vi "BlueSimpleReachTask catch trial.vi"() -> ()   [LabVIEW 2010]
uses:
  Controls/Bits to Write.ctl
panel:
  in  "Arm Freeze Counter":bool
  in  "Time to wait\nbefore treat \nArm freeze (S)":dbl
  in  "Catch probability":i32=5 min=0 max=100 step=1
  out "Catch Trial?":bool
  out "DO Task":refnum<k21>="BlueSimple_DO_All"
  out "DI Task":refnum<k21>="BlueSimple_DI"
  out "Exp correct":i32
  out "Record flag":bool
  in  "Recenter motor":bool
  in  "Override bumps":bool
  in  "Start bump timer?":bool
  in  "Trial type":u16(ring) items=["Allflash/sensory", "Precue/memory"]
  in  "DBS On?":bool
  in  "Home+target OK?":bool
  out "Exp reset":bool
  out "target set #":i32
  in  "duration (s)":dbl=0.18 format="%.4f"
  in  "Inter-pulse delay":cluster{"Fix":dbl, "Rnd":dbl}={"Fix"=0.0, "Rnd"=1.5} {"Rnd" format="%.4f"; "Fix" format="%_4g"}
  in  "Autofeed?":bool
  out "Just initialized\nhold loop?":bool
  in  "Home reward?":bool
  in  "Home reward":cluster{"Fix":dbl, "Rnd":dbl} {"Rnd" format="%.4f"; "Fix" format="%_4g"}
  in  "Override 4":bool caption="Override 1"
  in  "Override 3":bool caption="Override 1"
  in  "Override 2":bool=TRUE caption="Override 1"
  in  "Override 1":bool=TRUE
  in  "LED lines":T1={"LED1"=1, "LED2"=2, "LED3"=3, "LED4"=4}
  in  "LED1":i16=5
  in  "LED2":i16=6
  in  "LED3":i16=7
  in  "LED4":i16=8
  in  "Bump Parameters":T2={"Distance (deg)"=2.0, "Travel time (ms)"=500.0} {"Travel time (ms)" min=0.1 max=10000.0; "Distance (deg)" min=0.1}
  in  "Bump delay":cluster{"Fix":dbl, "Rnd":dbl}={"Fix"=2.0, "Rnd"=8.0} {"Rnd" format="%.4f"; "Fix" format="%_4g"}
  in  "Sine parameters":T3={"Frequency"=1.0, "Degrees\npk-pk"=8.0, "Cycles"=10000} {"Degrees\npk-pk" min=0.1 max=120.0; "Frequency" min=0.001 format="%#_4g"}
  in  "Home":bool
  in  "Bumps":bool
  in  "Sines?":bool
  out "target set size":i32
  out "# target sets":u16
  in  "# Cycles":i16=20
  out "Instruct duration":dbl format="%.4f"
  out "Pre-I hold":dbl format="%.4f"
  out "Touching target\nlast time?":bool
  in  "Rand/Seq?":bool=TRUE
  in  "Target set":i16[](array[ring]) items=["1", "2", "3", "4"]
  in  "Block":T4(array[cluster])
  in  "Settings In":T5={"Pre-I hold"={"Fixed (s)"=0.5, "Random (s)"=0.5}, "LED I duration"={"Fixed (s)"=0.5, "Random (s)"=0.0}, "All Flash?"=FALSE, "Pre-cue brightness"=0, "Post-I hold"={"Fixed (s)"=0.7, "Random (s)"=0.3}, "Post-I \nbounce-off"={"Fixed (s)"=0.3, "Random (s)"=0.0}, "Capture timeout"={"Fixed (s)"=1.5, "Random (s)"=0.0}, "Tone duration"={"Fixed (s)"=0.5, "Random (s)"=0.0}, "LED C duration"={"Fixed (s)"=0.5, "Random (s)"=0.0}, "Cue brightness"=0, "Hold duration"={"Fixed (s)"=0.3, "Random (s)"=0.0}, "Allowed\nbounce-off"={"Fixed (s)"=0.2, "Random (s)"=0.0}, "Post-capture brightness"=0, "Reward duration"={"Fixed (s)"=0.7, "Random (s)"=0.0}, "Intertrial interval"={"Fixed (s)"=0.5, "Random (s)"=0.0}, "Persistent Mode?"=FALSE, "Error bong?"=TRUE, "Critter"=0, "Blocks"=[], "Target set"=[], "Rand/Seq?"=TRUE, "Trial type"=0, "Sines?"=FALSE, "Bumps"=FALSE, "Sine parameters"={"Frequency"=0.25, "Degrees\npk-pk"=6.0, "Cycles"=10000}, "Bump timing"={"Fix"=2.0, "Rnd"=8.0}, "Bump Parameters"={"Distance (deg)"=2.0, "Travel time (ms)"=500.0}, "DBS On?"=FALSE, "Home reward?"=FALSE, "Home+target OK?"=FALSE} {"Bump Parameters"."Travel time (ms)" min=0.1 max=10000.0; "Bump Parameters"."Distance (deg)" min=0.1; "Bump timing"."Rnd" format="%.4f"; "Bump timing"."Fix" format="%_4g"; "Sine parameters"."Degrees\npk-pk" min=0.1 max=120.0; "Sine parameters"."Frequency" min=0.001 format="%#_4g"; "Trial type" items=["Allflash/sensory", "Precue/memory"]; "Target set" items=["1", "2", "3", "4"]; "Critter" items=["Mojo", "Smokey"]; "Post-I \nbounce-off"."Random (s)" format="%.4f"; "Post-I \nbounce-off"."Fixed (s)" format="%_4g"; "Allowed\nbounce-off"."Random (s)" format="%.4f"; "Allowed\nbounce-off"."Fixed (s)" format="%_4g"; "LED C duration"."Random (s)" format="%.4f"; "LED C duration"."Fixed (s)" format="%.4f"; "Capture timeout"."Random (s)" format="%.4f"; "Capture timeout"."Fixed (s)" format="%.4f"; "Post-I hold"."Random (s)" format="%.4f"; "Post-I hold"."Fixed (s)" format="%.4f"; "Hold duration"."Random (s)" format="%.4f"; "Hold duration"."Fixed (s)" format="%_4g"; "Intertrial interval"."Random (s)" format="%.4f"; "Intertrial interval"."Fixed (s)" format="%.4f"; "Reward duration"."Random (s)" format="%.4f"; "Reward duration"."Fixed (s)" format="%.4f"; "LED I duration"."Random (s)" format="%.4f"; "LED I duration"."Fixed (s)" format="%.4f"; "Tone duration"."Random (s)" format="%.4f"; "Tone duration"."Fixed (s)" format="%.4f"; "Pre-I hold"."Random (s)" format="%.4f"; "Pre-I hold"."Fixed (s)" format="%_4g"}
  in  "pause":bool
  out "Assign settings":bool
  out "current path":path
  out "next trial path":path
  in  "Critter":u16(ring) items=["Mojo", "Smokey", "Blue", "Odo", "Monk 5", "Monk 6", "Monk 7", "Monk 8", "Monk 9", "Monk 10"]
  out "Total incorrect":i32
  in  "Write Settings":bool
  in  "Read Settings":bool
  in  "All Flash?":bool
  in  "Post-capture brightness":i16 caption="Brightness"
  in  "Cue brightness":i16=6 caption="Brightness"
  in  "Pre-cue brightness":i16 caption="Brightness"
  out "Total correct":i32
  out "Total %":dbl
  out "Total trials":i32
  in  "Error\nbong?":bool=TRUE
  out "TS Home":bool
  out "TS 4":bool
  out "TS 3":bool
  out "TS 2":bool
  out "TS 1":bool
  out "Waveform Chart":T6(graph)
  out "Block trials":i32
  out "Block %":dbl
  in  "Reset\ncounters":bool
  in  "Post-I \nbounce-off":cluster{"Fix":dbl, "Rnd":dbl}={"Fix"=0.3, "Rnd"=0.0} caption="Allowed\nbounce-off" {"Rnd" format="%.4f"; "Fix" format="%_4g"}
  out "Exp trials":i32
  out "Exp %":dbl
  in  "Touch lines":T7={"Home touch"=0, "Touch 1"=1, "Touch 2"=2, "Touch 3"=3, "Touch 4"=4}
  out "Current stage":T8(ring)
  in  "Allowed\nbounce-off":cluster{"Fix":dbl, "Rnd":dbl}={"Fix"=0.2, "Rnd"=0.0} {"Rnd" format="%.4f"; "Fix" format="%_4g"}
  in  "LED C duration":cluster{"Fix":dbl, "Rnd":dbl}={"Fix"=0.5, "Rnd"=0.0} caption="LED duration" {"Rnd" format="%.4f"; "Fix" format="%.4f"}
  in  "Capture timeout":cluster{"Fix":dbl, "Rnd":dbl}={"Fix"=1.5, "Rnd"=0.0} caption="Response time" {"Rnd" format="%.4f"; "Fix" format="%.4f"}
  in  "Post-I hold":cluster{"Fix":dbl, "Rnd":dbl}={"Fix"=0.5, "Rnd"=0.5} {"Rnd" format="%.4f"; "Fix" format="%.4f"}
  out "Last trial successful?":bool
  in  "Persistent\n Mode?":bool
  in  "Touch 4":i16=4
  in  "Touch 3":i16=3
  in  "Touch 2":i16=2
  in  "Touch 1":i16=1
  in  "Home touch":i16
  in  "Hold duration":cluster{"Fix":dbl, "Rnd":dbl}={"Fix"=0.2, "Rnd"=0.0} {"Rnd" format="%.4f"; "Fix" format="%_4g"}
  out "Target":i16
  in  "stop":bool
  in  "device":i16=1
  in  "line direction map":i32=2147483616 format="%.0b"
  out "DIGIO task ID":u32 format="%.0x"
  out "error out":errorcluster
  in  "Intertrial interval":cluster{"Fix":dbl, "Rnd":dbl}={"Fix"=0.5, "Rnd"=0.0} {"Rnd" format="%.4f"; "Fix" format="%.4f"}
  in  "Reward duration":cluster{"Fix":dbl, "Rnd":dbl}={"Fix"=0.38, "Rnd"=0.1} {"Rnd" format="%.4f"; "Fix" format="%.4f"}
  in  "LED I duration":cluster{"Fix":dbl, "Rnd":dbl}={"Fix"=0.5, "Rnd"=0.0} caption="LED duration" {"Rnd" format="%.4f"; "Fix" format="%.4f"}
  in  "Tone duration":cluster{"Fix":dbl, "Rnd":dbl}={"Fix"=0.5, "Rnd"=0.0} {"Rnd" format="%.4f"; "Fix" format="%.4f"}
  in  "Pre-I hold":cluster{"Fix":dbl, "Rnd":dbl}={"Fix"=0.5, "Rnd"=0.5} {"Rnd" format="%.4f"; "Fix" format="%_4g"}
  # "Auto-feed"
  # "DBS"
  # "Pre-\ninstruction\nhold"
  # "Post-\ninstruction\nhold"
  # "Instruction"
  # "Target capture"
  # "Target hold"
  # "Reward"
  # "Intertrial"
  # "Motor"
  # "Override"
  # "+"
  # "+"
  # "+"
  # "Pre-\ninstruction\nhold"
  # "Instruction"
  # "Post-\ninstruction\nhold"
  # "Target capture"
  # "Target hold"
  # "Reward"
  # "Intertrial"
  # "+"
  # "+"
  # "+"
  # "+"
  # "+"
  # "+"
  # "+"
  # "+"
  # "+"
  # "+"
  # "+"
  # "+"
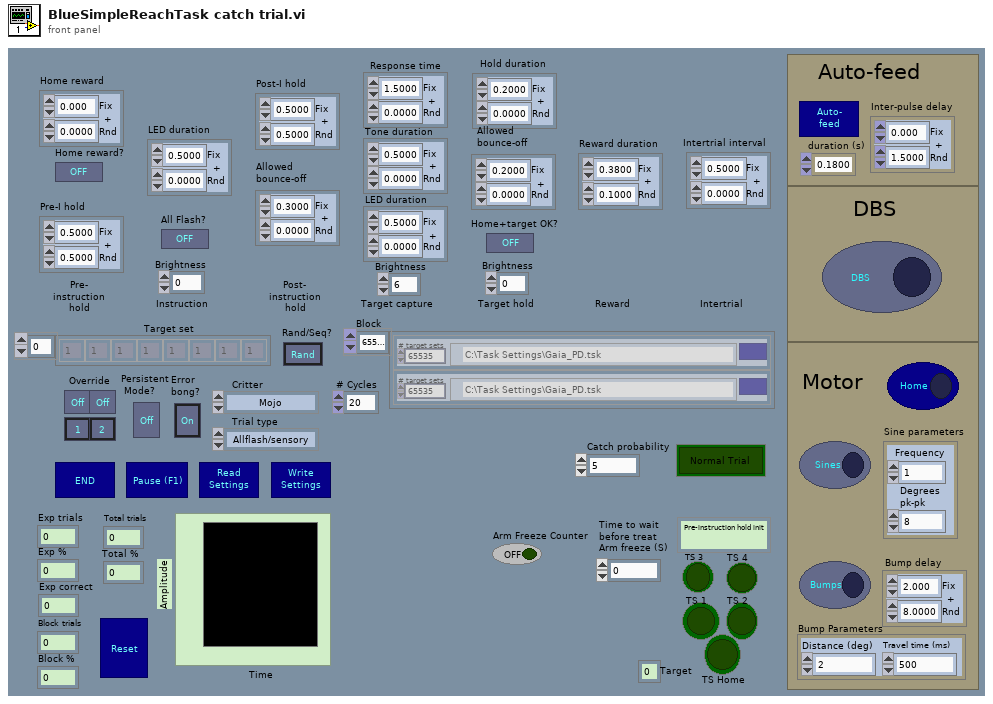
[diagram p1: front panel]
types:
  T1 = cluster{"LED1":i16, "LED2":i16, "LED3":i16, "LED4":i16}
  T2 = cluster{"Distance (deg)":dbl, "Travel time (ms)":dbl}
  T3 = cluster{"Frequency":dbl, "Degrees\npk-pk":dbl, "Cycles":i16}
  T4 = cluster{"Settings file":path, "# target sets":u16}[]
  T5 = cluster{"Pre-I hold":cluster{"Fixed (s)":dbl, "Random (s)":dbl}, "LED I duration":cluster{"Fixed (s)":dbl, "Random (s)":dbl}, "All Flash?":bool, "Pre-cue brightness":i16, "Post-I hold":cluster{"Fixed (s)":dbl, "Random (s)":dbl}, "Post-I \nbounce-off":cluster{"Fixed (s)":dbl, "Random (s)":dbl}, "Capture timeout":cluster{"Fixed (s)":dbl, "Random (s)":dbl}, "Tone duration":cluster{"Fixed (s)":dbl, "Random (s)":dbl}, "LED C duration":cluster{"Fixed (s)":dbl, "Random (s)":dbl}, "Cue brightness":i16, "Hold duration":cluster{"Fixed (s)":dbl, "Random (s)":dbl}, "Allowed\nbounce-off":cluster{"Fixed (s)":dbl, "Random (s)":dbl}, "Post-capture brightness":i16, "Reward duration":cluster{"Fixed (s)":dbl, "Random (s)":dbl}, "Intertrial interval":cluster{"Fixed (s)":dbl, "Random (s)":dbl}, "Persistent Mode?":bool, "Error bong?":bool, "Critter":u16, "Blocks":cluster{"Settings file":path, "# target sets":dbl}[], "Target set":i16[], "Rand/Seq?":bool, "Trial type":u16, "Sines?":bool, "Bumps":bool, "Sine parameters":cluster{"Frequency":dbl, "Degrees\npk-pk":dbl, "Cycles":i16}, "Bump timing":cluster{"Fix":dbl, "Rnd":dbl}, "Bump Parameters":cluster{"Distance (deg)":dbl, "Travel time (ms)":dbl}, "DBS On?":bool, "Home reward?":bool, "Home+target OK?":bool}
  T6 = cluster{"Segment Percentage":dbl, "Total % correct":dbl}
  T7 = cluster{"Home touch":i16, "Touch 1":i16, "Touch 2":i16, "Touch 3":i16, "Touch 4":i16}
  T8 = enum16{"Pre-instruction hold init", "Pre-instruction hold", "Instruction init", "Instruction", "Post-instruction hold init", "Post-instruction hold", "Target capture init", "Target capture", "Target hold init", "Target hold", "Reward stage", "Intertrial"}
  T9 = typedef "Bits to Write.ctl" = enum16{"LED 1 on", "LED 1 off", "LED 2 on", "LED 2 off", "LED 3 on", "LED 3 off", "LED 4 on", "LED 4 off", "All LEDs on", "All LEDs off", "In trial on", "In trial off", "Buzzer on", "Buzzer off", "Reward on", "Reward off", "Target number", "Trial type preQ on", "Trial type preQ off", "Error on", "Error off", "Trial number", "DBS on", "DBS off", "Sine on", "Sine off", "All Bits On", "All Bits Off", "Init", "Specify mask/pattern"}
  T10 = enum16{"Reset", "Increment", "Reset for exp", "Initialize"}
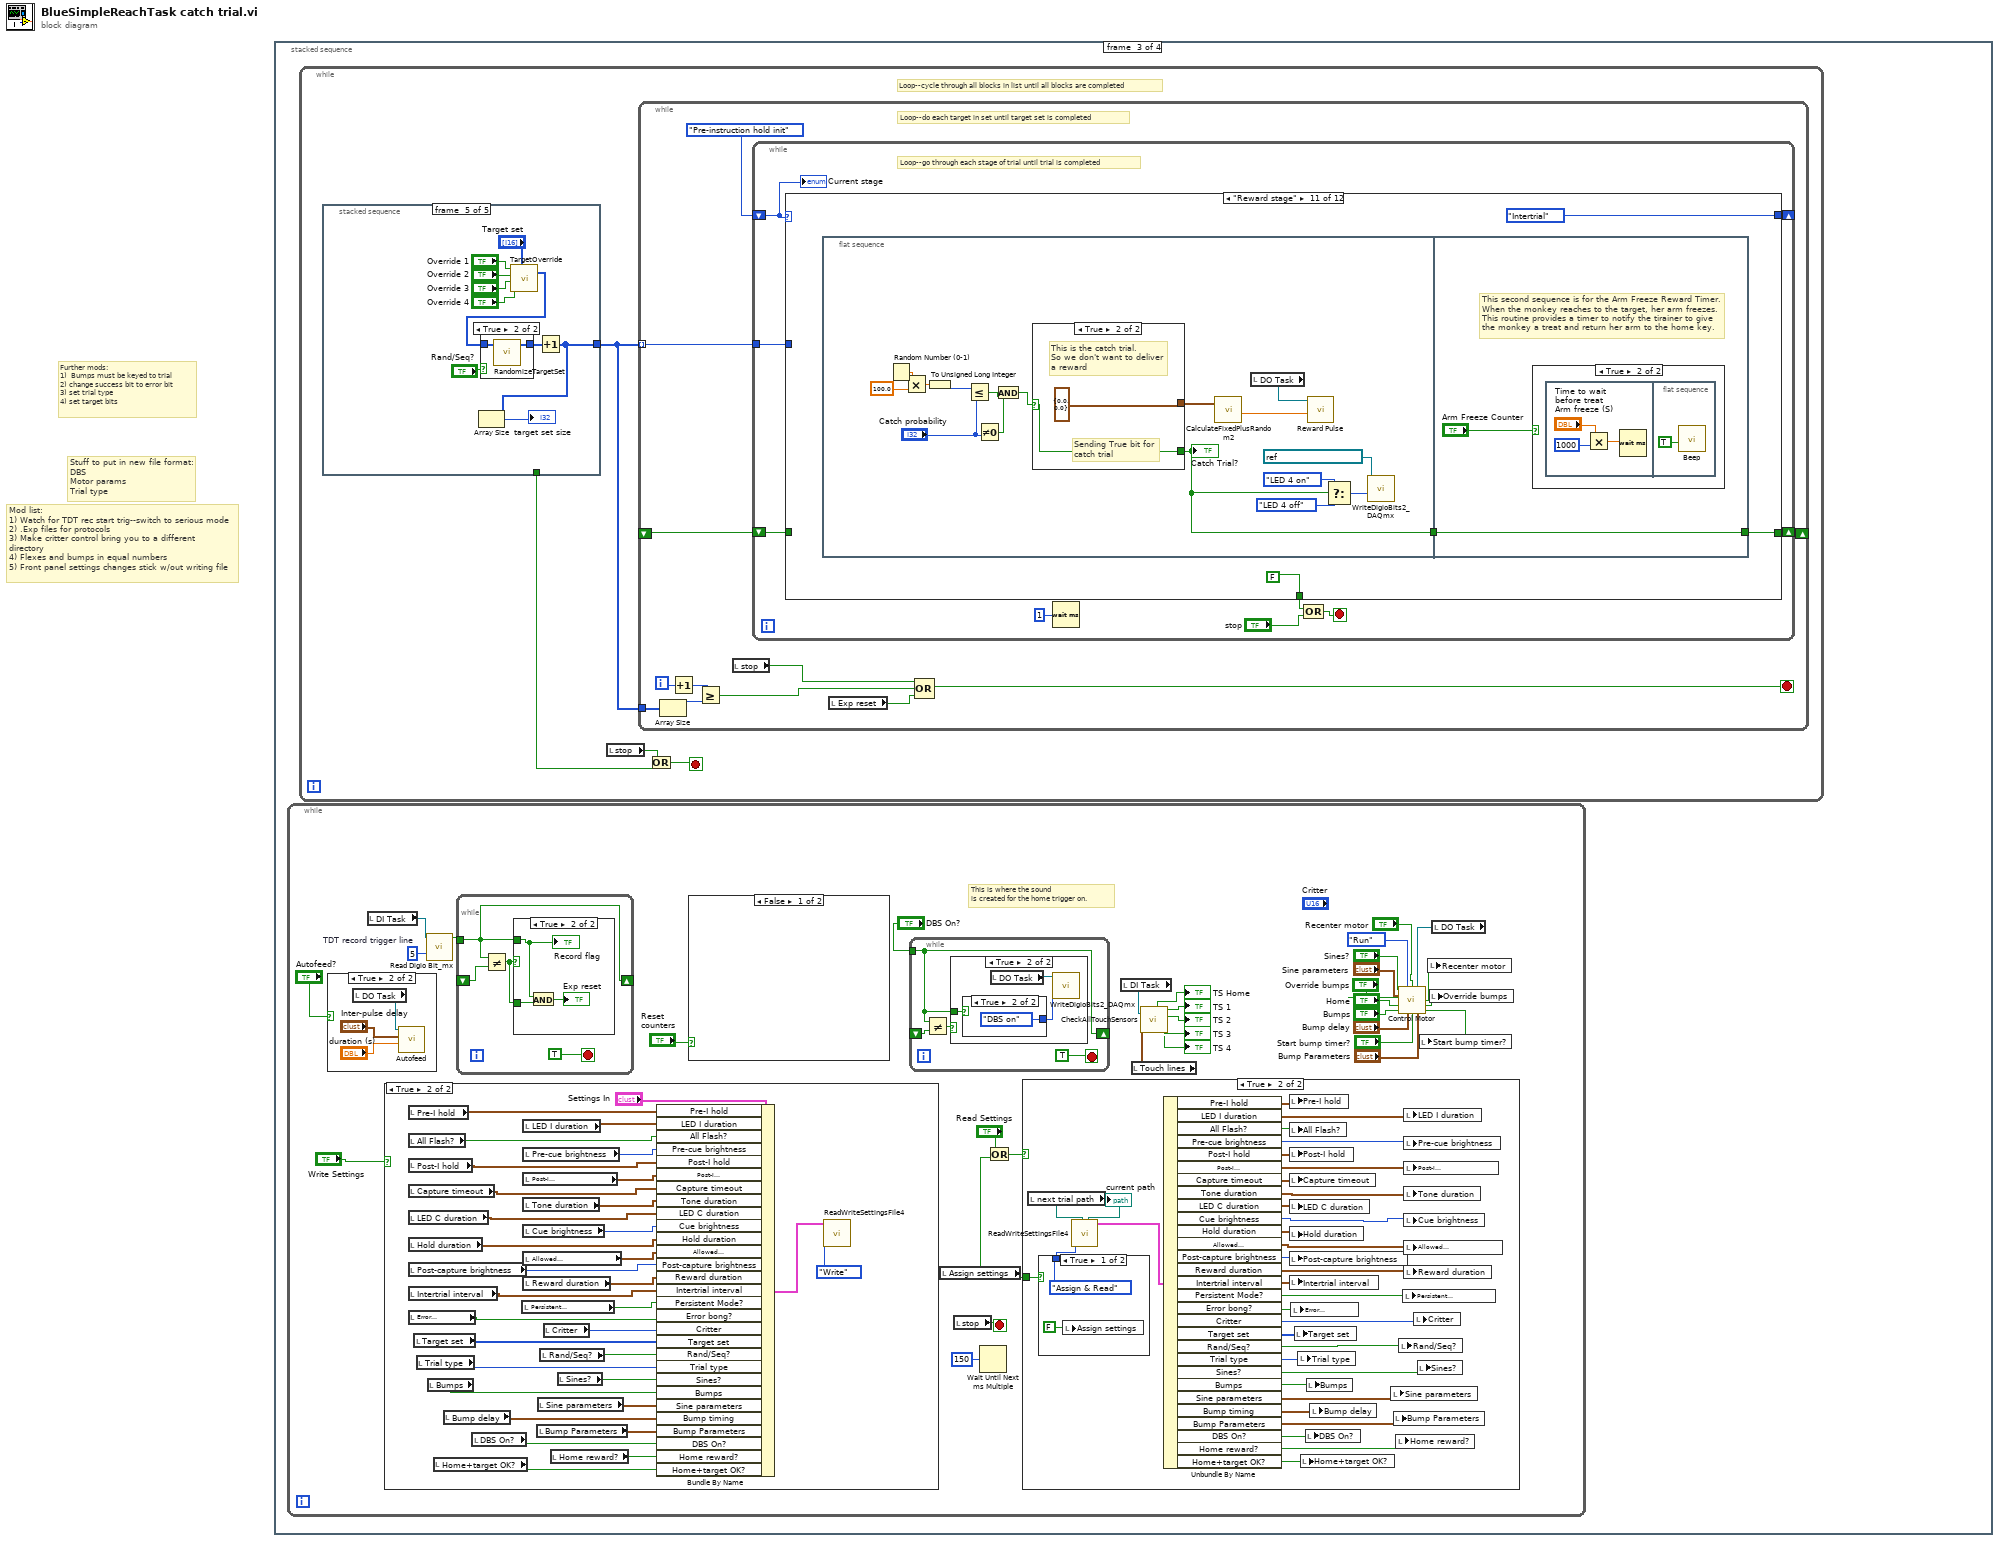
[diagram p0: block diagram]
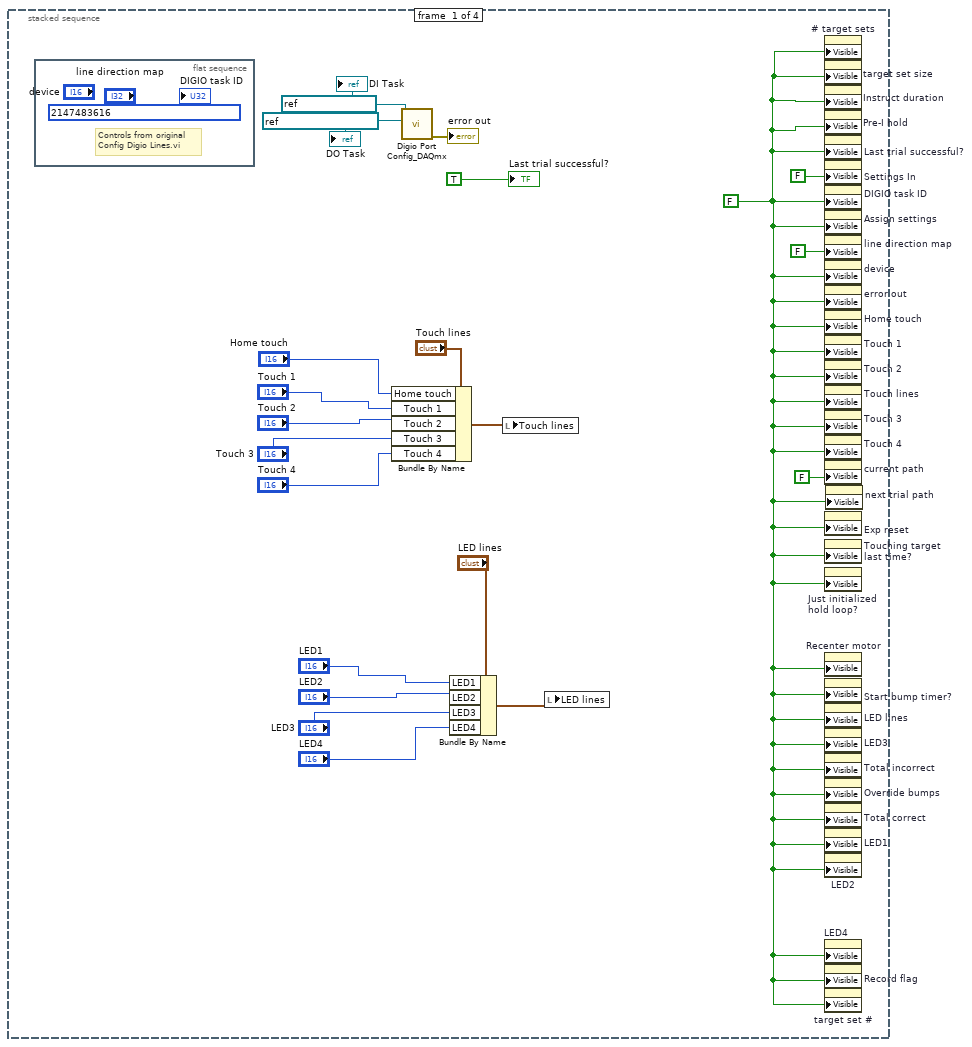
[diagram p2: hidden frame]
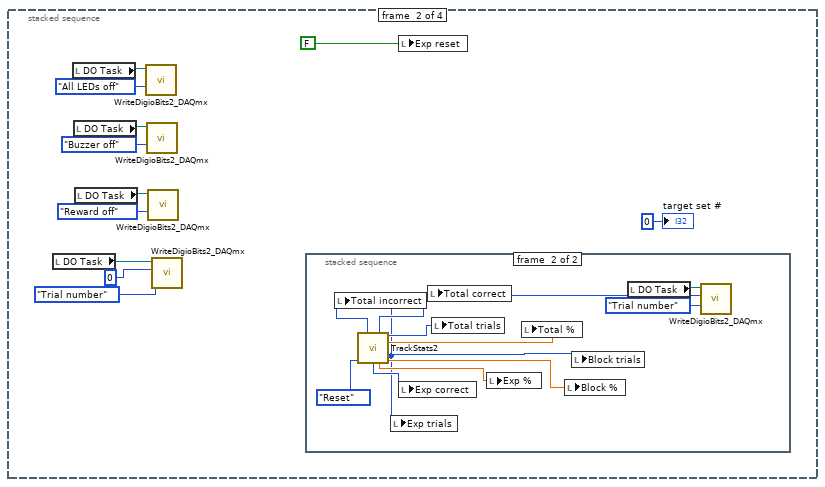
[diagram p3: hidden frame]
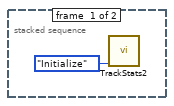
[diagram p4: hidden frame]
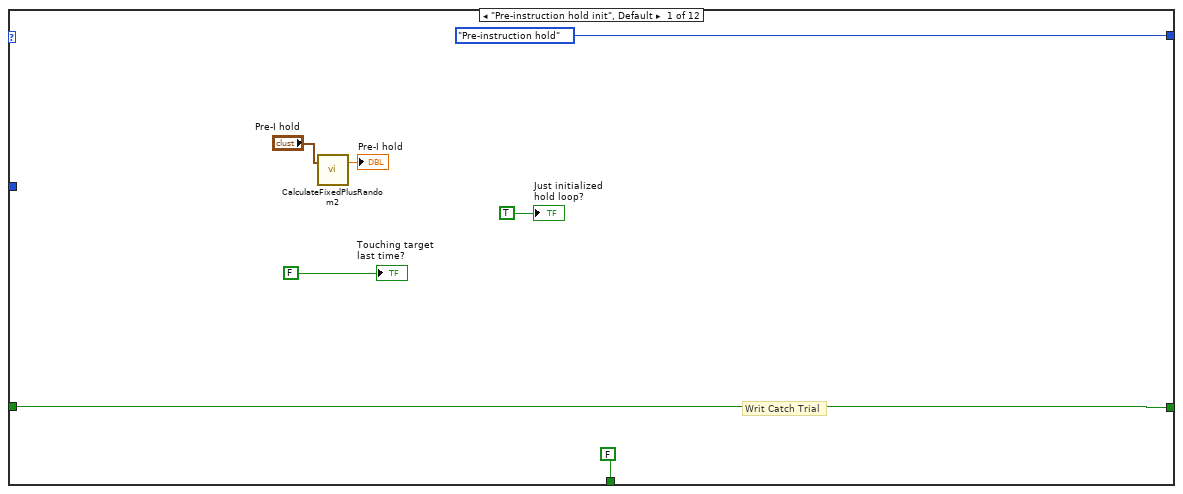
[diagram p5: hidden frame]
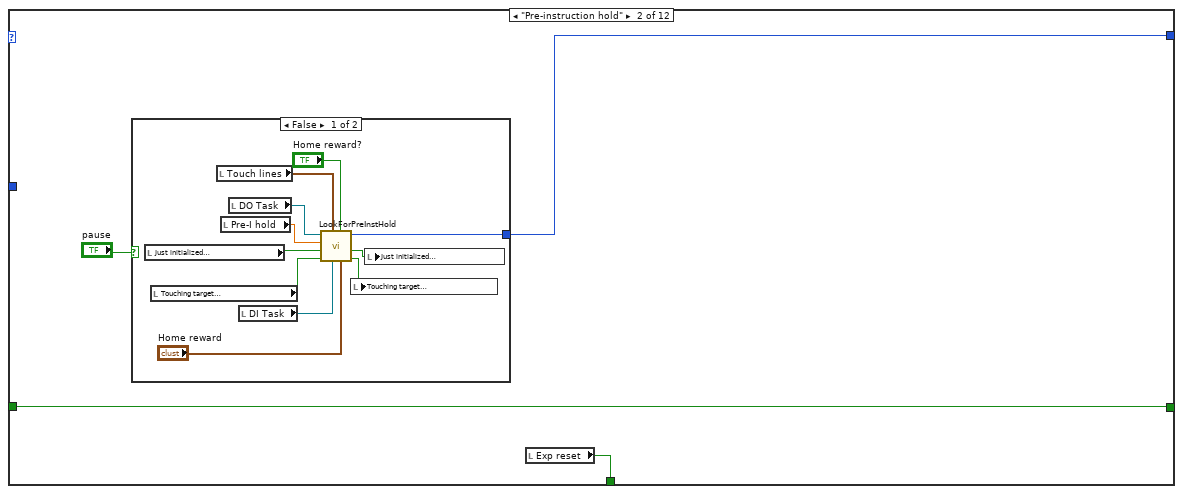
[diagram p6: hidden frame]
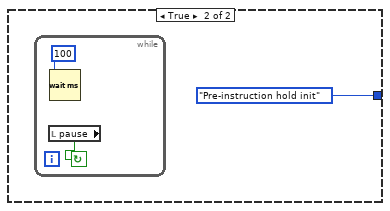
[diagram p7: hidden frame]
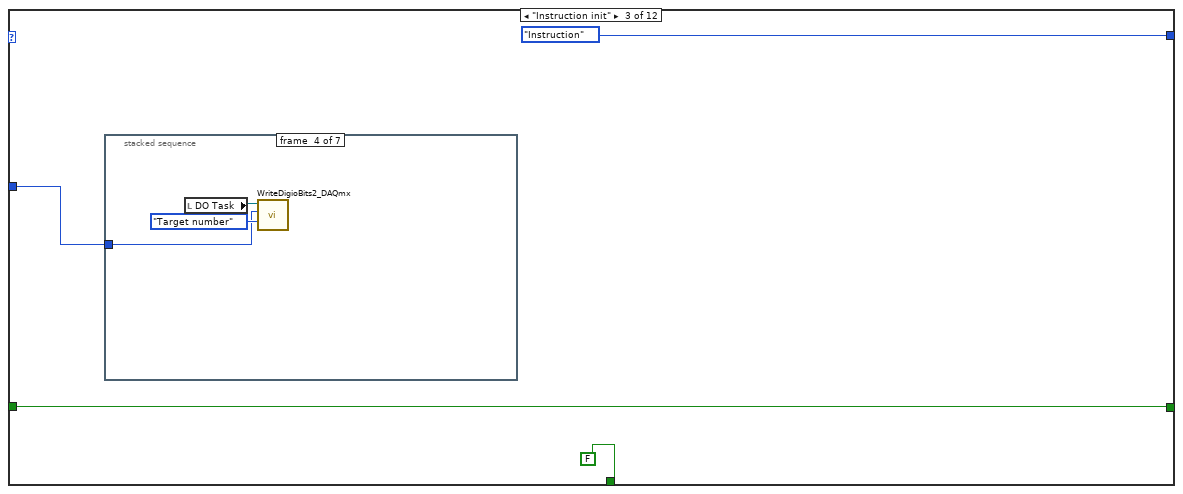
[diagram p8: hidden frame]
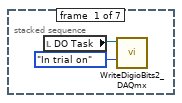
[diagram p9: hidden frame]
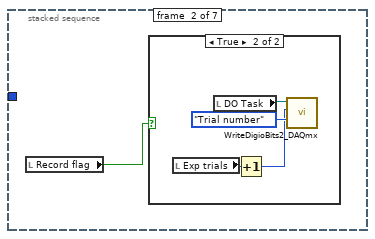
[diagram p10: hidden frame]
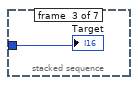
[diagram p12: hidden frame]
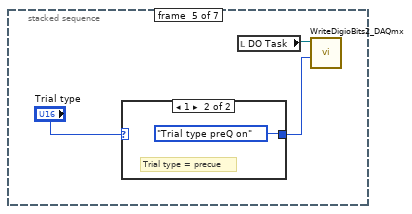
[diagram p13: hidden frame]
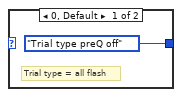
[diagram p14: hidden frame]
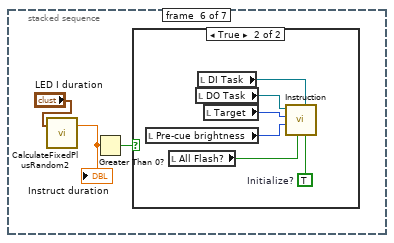
[diagram p15: hidden frame]
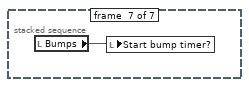
[diagram p17: hidden frame]
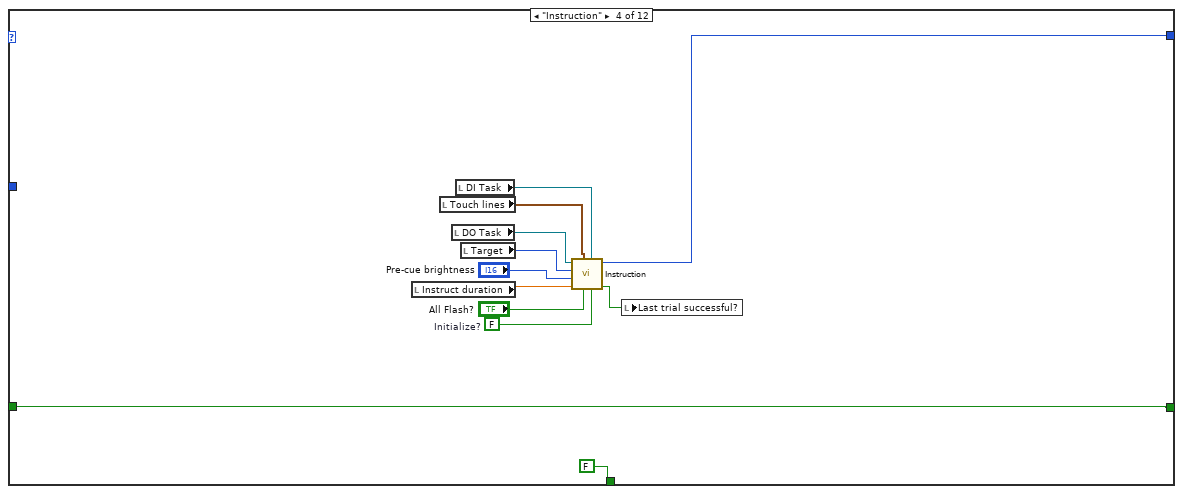
[diagram p18: hidden frame]
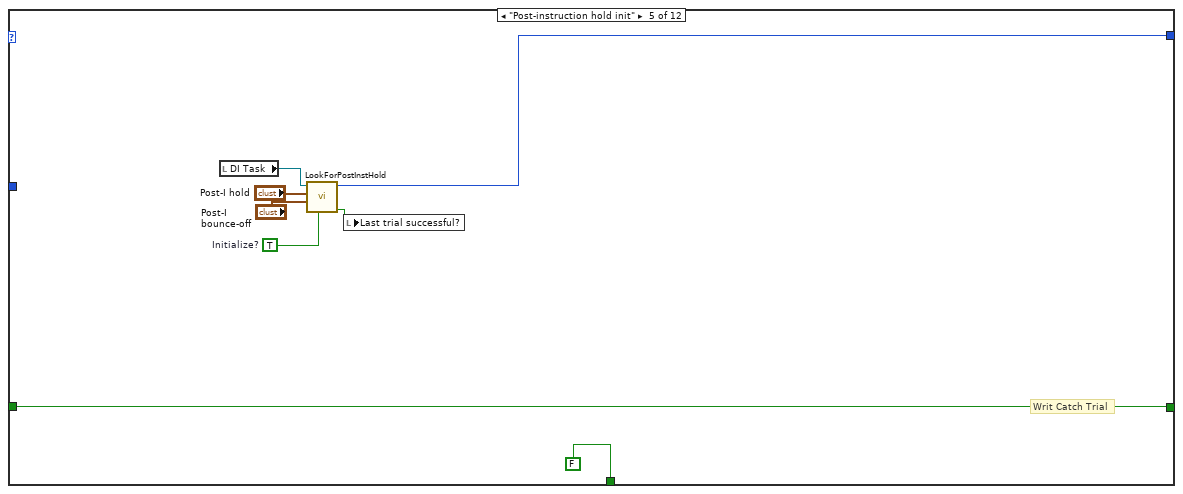
[diagram p19: hidden frame]
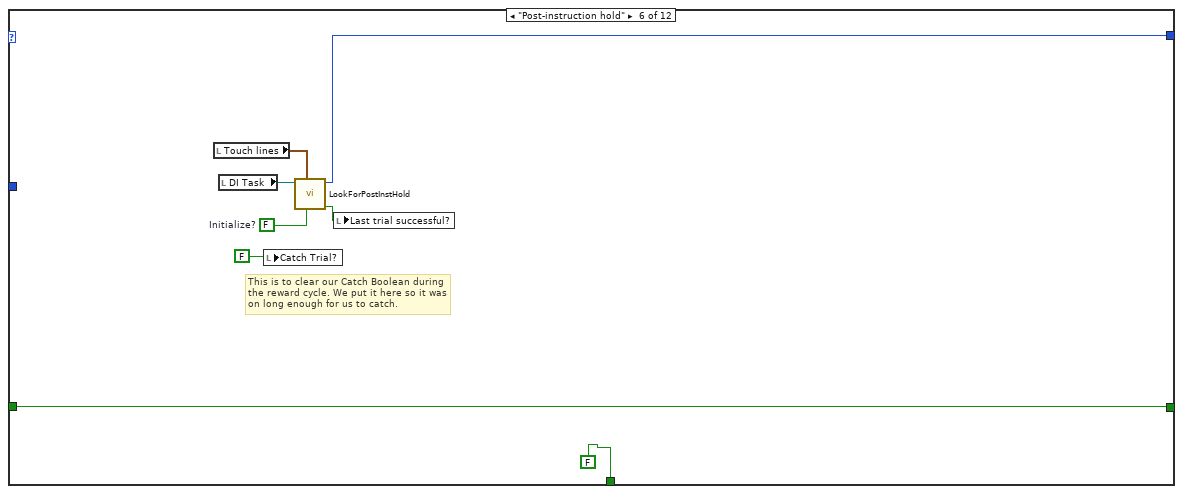
[diagram p20: hidden frame]
diagram:
  # "Stuff to put in new file format:\nDBS\nMotor params\nTrial type"
  # "Further mods:\n1)  Bumps must be keyed to trial\n2) change success bit to error bit\n3) set trial type\n4) set target bits"
  # "Mod list:\n1) Watch for TDT rec start trig--switch to serious mode\n2) .Exp files for protocols\n3) Make critter control bring you to a different directory\n4) Flexes and bumps in equal numbers\n5) Front panel settings changes stick w/out writing file"
  n1 = stacked-sequence {
    frame #0 {
      w2 = refnum<k21> "BlueSimple_DO_All" ("DO Task")
      w3 = refnum<k21> "BlueSimple_DI" ("DI Task")
      w4 = FALSE ("Persistent Mode?")
      n2 = flat-sequence {
        frame #0 {
          (unwired) 2147483616 ("line direction map")
          # "Controls from original\nConfig Digio Lines.vi"
        }
      }
      n3 = Bundle By Name(cluster="Touch lines", "Home touch"="Home touch", "Touch 1"="Touch 1", "Touch 2"="Touch 2", "Touch 3"="Touch 3", "Touch 4"="Touch 4") -> (w20:T7)
      n4 = call "Digio Port Config_DAQmx.vi"("DO Task"=w2, "DI Task"=w3) -> ("error out"=→"error out":errorcluster)  [unwired: 7 in]
      n5 = Bundle By Name(cluster="LED lines", "LED1"="LED1", "LED2"="LED2", "LED3"="LED3", "LED4"="LED4") -> (w8:T1)
      n6 = local write "Touch lines"(w20) -> ()
      n7 = local write "LED lines"(w8) -> ()
      n8 = property on="# target sets" class="DigNum (strict)"("Visible"=w4) -> ()  [unwired: 2 in, 2 out]
      n9 = property on="target set size" class="DigNum (strict)"("Visible"=w4) -> ()  [unwired: 2 in, 2 out]
      n10 = property on="Instruct duration" class="DigNum (strict)"("Visible"=w4) -> ()  [unwired: 2 in, 2 out]
      n11 = property on="Pre-I hold" class="DigNum (strict)"("Visible"=w4) -> ()  [unwired: 2 in, 2 out]
      n12 = property on="Last trial successful?" class="Bool (strict)"("Visible"=w4) -> ()  [unwired: 2 in, 2 out]
      n13 = property on="Settings In" class="Clust (strict)"("Visible"=FALSE) -> ()  [unwired: 2 in, 2 out]
      n14 = property on="DIGIO task ID" class="DigNum (strict)"("Visible"=w4) -> ()  [unwired: 2 in, 2 out]
      n15 = property on="Assign settings" class="Bool (strict)"("Visible"=w4) -> ()  [unwired: 2 in, 2 out]
      n16 = property on="line direction map" class="DigNum (strict)"("Visible"=FALSE) -> ()  [unwired: 2 in, 2 out]
      n17 = property on="device" class="DigNum (strict)"("Visible"=w4) -> ()  [unwired: 2 in, 2 out]
      n18 = property on="error out" class="Clust (strict)"("Visible"=w4) -> ()  [unwired: 2 in, 2 out]
      n19 = property on="Home touch" class="DigNum (strict)"("Visible"=w4) -> ()  [unwired: 2 in, 2 out]
      n20 = property on="Touch 1" class="DigNum (strict)"("Visible"=w4) -> ()  [unwired: 2 in, 2 out]
      n21 = property on="Touch 2" class="DigNum (strict)"("Visible"=w4) -> ()  [unwired: 2 in, 2 out]
      n22 = property on="Touch lines" class="Clust (strict)"("Visible"=w4) -> ()  [unwired: 2 in, 2 out]
      n23 = property on="Touch 3" class="DigNum (strict)"("Visible"=w4) -> ()  [unwired: 2 in, 2 out]
      n24 = property on="Touch 4" class="DigNum (strict)"("Visible"=w4) -> ()  [unwired: 2 in, 2 out]
      n25 = property on="current path" class="Path"("Visible"=FALSE) -> ()  [unwired: 2 in, 2 out]
      n26 = property on="Exp reset" class="Bool (strict)"("Visible"=w4) -> ()  [unwired: 2 in, 2 out]
      n27 = property on="Touching target\nlast time?" class="Bool (strict)"("Visible"=w4) -> ()  [unwired: 2 in, 2 out]
      n28 = property on="Just initialized\nhold loop?" class="Bool (strict)"("Visible"=w4) -> ()  [unwired: 2 in, 2 out]
      n29 = property on="Recenter motor" class="Bool (strict)"("Visible"=w4) -> ()  [unwired: 2 in, 2 out]
      n30 = property on="Start bump timer?" class="Bool (strict)"("Visible"=w4) -> ()  [unwired: 2 in, 2 out]
      n31 = property on="LED lines" class="Clust (strict)"("Visible"=w4) -> ()  [unwired: 2 in, 2 out]
      n32 = property on="LED3" class="DigNum (strict)"("Visible"=w4) -> ()  [unwired: 2 in, 2 out]
      n33 = property on="Total incorrect" class="DigNum (strict)"("Visible"=w4) -> ()  [unwired: 2 in, 2 out]
      n34 = property on="Override bumps" class="Bool (strict)"("Visible"=w4) -> ()  [unwired: 2 in, 2 out]
      n35 = property on="Total correct" class="DigNum (strict)"("Visible"=w4) -> ()  [unwired: 2 in, 2 out]
      n36 = property on="LED1" class="DigNum (strict)"("Visible"=w4) -> ()  [unwired: 2 in, 2 out]
      n37 = property on="LED2" class="DigNum (strict)"("Visible"=w4) -> ()  [unwired: 2 in, 2 out]
      n38 = property on="LED4" class="DigNum (strict)"("Visible"=w4) -> ()  [unwired: 2 in, 2 out]
      n39 = property on="Record flag" class="Bool (strict)"("Visible"=w4) -> ()  [unwired: 2 in, 2 out]
      n40 = property on="target set #" class="DigNum (strict)"("Visible"=w4) -> ()  [unwired: 2 in, 2 out]
      n41 = property on="next trial path" class="Path"("Visible"=w4) -> ()  [unwired: 2 in, 2 out]
      "Last trial successful?" <- TRUE ("Persistent Mode?")
      "DI Task" <- w3
      "DO Task" <- w2
    }
    frame #1 {
      n42 = local read "DO Task"() -> (w30:refnum<k21>)
      n43 = local read "DO Task"() -> (w23:refnum<k21>)
      n44 = local read "DO Task"() -> (w24:refnum<k21>)
      n45 = local read "DO Task"() -> (w26:refnum<k21>)
      n46 = call "WriteDigioBits2_DAQmx.vi"("Bits to write"=Bits_to_Write."All LEDs off", "DO Task"=w23) -> ()  [unwired: 9 in, 1 out]
      n47 = call "WriteDigioBits2_DAQmx.vi"("Bits to write"=Bits_to_Write."Buzzer off", "DO Task"=w24) -> ()  [unwired: 9 in, 1 out]
      n48 = call "WriteDigioBits2_DAQmx.vi"("Bits to write"=Bits_to_Write."Reward off", "DO Task"=w26) -> ()  [unwired: 9 in, 1 out]
      n49 = call "WriteDigioBits2_DAQmx.vi"("Bits to write"=Bits_to_Write."Trial number", "Number"=u32 0, "DO Task"=w30) -> ()  [unwired: 8 in, 1 out]
      n50 = stacked-sequence {
        frame #0 {
          n51 = call "TrackStats2.vi"("Command"=T10."Initialize") -> ()  [unwired: 6 in, 9 out]
        }
        frame #1 {
          n52 = call "TrackStats2.vi"("Command"=T10."Reset") -> ("Total incorrect"=w45:i32, "Total correct"=w44:i32, "# total trials"=w43:i32, "Total % correct"=w42:dbl, "Segment trials"=w38:i32, "Experiment trials"=w34:i32, "Experiment correct"=w37:i32, "Experiment %"=w40:dbl, "Segment Percentage"=w41:dbl)  [unwired: 6 in]
          n53 = local write "Total incorrect"(w45) -> ()
          n54 = local write "Exp trials"(w34) -> ()
          n55 = local write "Exp correct"(w37) -> ()
          n56 = local write "Total correct"(w44) -> ()
          n57 = local write "Total trials"(w43) -> ()
          n58 = local write "Exp %"(w40) -> ()
          n59 = local write "Total %"(w42) -> ()
          n60 = local write "Block %"(w41) -> ()
          n61 = local write "Block trials"(w38) -> ()
          n62 = local read "DO Task"() -> (w36:refnum<k21>)
          n63 = call "WriteDigioBits2_DAQmx.vi"("Bits to write"=Bits_to_Write."Trial number", "Number"=w34, "DO Task"=w36) -> ()  [unwired: 8 in, 1 out]
        }
      }
      n64 = local write "Exp reset"(FALSE ("Exp reset")) -> ()
      "target set #" <- 0 ("target set #")
    }
    frame #2 {
      n65 = while {
        stop <- w334 stop-if-true
        w305 = i16 5  # TDT record trigger line
        # "This is where the sound\nis created for the home trigger on."
        n66 = case shown="True" "Autofeed?" {
          frame False {
          }
          frame True {
            n67 = local read "DO Task"() -> (w344:refnum<k21>)
            n68 = call "Autofeed.vi"("duration"="duration (s)", "Auto-feed"="Inter-pulse delay", "DO Task"=w344) -> ()  [unwired: 4 in]
          }
        }
        n69 = local read "DI Task"() -> (w304:refnum<k21>)
        n70 = case shown="True" "Write Settings" {
          frame False {
          }
          frame True {
            n71 = local read "Pre-I hold"() -> (w385:cluster{"Fix":dbl, "Rnd":dbl})
            n72 = local read "All Flash?"() -> (w383:bool)
            n73 = local read "Post-I hold"() -> (w381:cluster{"Fix":dbl, "Rnd":dbl})
            n74 = local read "Capture timeout"() -> (w379:cluster{"Fix":dbl, "Rnd":dbl})
            n75 = local read "LED C duration"() -> (w377:cluster{"Fix":dbl, "Rnd":dbl})
            n76 = local read "Hold duration"() -> (w375:cluster{"Fix":dbl, "Rnd":dbl})
            n77 = local read "Post-capture brightness"() -> (w373:i16)
            n78 = local read "Intertrial interval"() -> (w371:cluster{"Fix":dbl, "Rnd":dbl})
            n79 = local read "Error\nbong?"() -> (w369:bool)
            n80 = local read "Target set"() -> (w365:i16[])
            n81 = local read "Trial type"() -> (w362:u16)
            n82 = local read "Bumps"() -> (w360:bool)
            n83 = local read "Home+target OK?"() -> (w354:bool)
            n84 = local read "Bump delay"() -> (w358:cluster{"Fix":dbl, "Rnd":dbl})
            n85 = local read "DBS On?"() -> (w356:bool)
            n86 = local read "Persistent\n Mode?"() -> (w370:bool)
            n87 = local read "LED I duration"() -> (w384:cluster{"Fix":dbl, "Rnd":dbl})
            n88 = local read "Pre-cue brightness"() -> (w382:i16)
            n89 = local read "Post-I \nbounce-off"() -> (w380:cluster{"Fix":dbl, "Rnd":dbl})
            n90 = local read "Tone duration"() -> (w378:cluster{"Fix":dbl, "Rnd":dbl})
            n91 = local read "Cue brightness"() -> (w376:i16)
            n92 = local read "Allowed\nbounce-off"() -> (w374:cluster{"Fix":dbl, "Rnd":dbl})
            n93 = local read "Reward duration"() -> (w372:cluster{"Fix":dbl, "Rnd":dbl})
            n94 = local read "Bump Parameters"() -> (w357:T2)
            n95 = local read "Sine parameters"() -> (w359:T3)
            n96 = local read "Rand/Seq?"() -> (w364:bool)
            n97 = local read "Critter"() -> (w366:u16)
            n98 = local read "Home reward?"() -> (w355:bool)
            n99 = local read "Sines?"() -> (w361:bool)
            n100 = Bundle By Name(cluster="Settings In", "Pre-I hold"=w385, "LED I duration"=w384, "All Flash?"=w383, "Pre-cue brightness"=w382, "Post-I hold"=w381, "Post-I \nbounce-off"=w380, "Capture timeout"=w379, "Tone duration"=w378, "LED C duration"=w377, "Cue brightness"=w376, "Hold duration"=w375, "Allowed\nbounce-off"=w374, "Post-capture brightness"=w373, "Reward duration"=w372, "Intertrial interval"=w371, "Persistent Mode?"=w370, "Error bong?"=w369, "Critter"=w366, "Target set"=w365, "Rand/Seq?"=w364, "Trial type"=w362, "Sines?"=w361, "Bumps"=w360, "Sine parameters"=w359, "Bump timing"=w358, "Bump Parameters"=w357, "DBS On?"=w356, "Home reward?"=w355, "Home+target OK?"=w354) -> (w363:T5)
            n101 = call "ReadWriteSettingsFile4.vi"("Read/write"=enum16{"Query & Read", "Assign & Read", "Write"}."Write", "Settings In"=w363) -> ()  [unwired: 4 in, 4 out]
          }
        }
        n102 = call "Read Digio Bit_mx.vi"("line"=w305, "DI Task"=w304) -> ("line state"=w303:bool)  [unwired: 7 in, 1 out]
        n103 = while {
          tunnel: w303 -> [w348]
          shift-right: [w348] -> _
          shift-left: _ -> [w349]
          stop <- TRUE stop-if-true
          n104 = Not Equal?(x=w348, y=w349) -> (x != y?=w347:bool)
          n105 = case shown="True" w347 {
            tunnel: w348 -> [_ w351]
            tunnel: w347 -> [_ w352]
            frame False {
            }
            frame True {
              n106 = And(x=w351, y=w352) -> (x .and. y?=→"Exp reset":bool)
              "Record flag" <- w351
            }
          }
        }
        n107 = case shown="False" "Reset\ncounters" {
          frame False {
          }
          frame True {
            n108 = call "TrackStats2.vi"("Command"=T10."Reset") -> ("Total incorrect"=w431:i32, "Total correct"=w430:i32, "# total trials"=w429:i32, "Total % correct"=w428:dbl, "Segment trials"=w427:i32, "Experiment trials"=w424:i32, "Experiment %"=w425:dbl, "Segment Percentage"=w426:dbl)  [unwired: 6 in, 1 out]
            n109 = local write "Total incorrect"(w431) -> ()
            n110 = local write "Total correct"(w430) -> ()
            n111 = local write "Exp trials"(w424) -> ()
            n112 = local write "Exp %"(w425) -> ()
            n113 = local write "Block %"(w426) -> ()
            n114 = local write "Block trials"(w427) -> ()
            n115 = local write "Total trials"(w429) -> ()
            n116 = local write "Total %"(w428) -> ()
          }
        }
        n117 = while {
          shift-right: [w336] -> _
          shift-left: _ -> [w337]
          tunnel: "DBS On?" -> [w336]
          stop <- TRUE stop-if-true
          n118 = Not Equal?(x=w336, y=w337) -> (x != y?=w335:bool)
          n119 = case shown="True" w335 {
            tunnel: w336 -> [_ w341]
            frame False {
            }
            frame True {
              n120 = case shown="True" w341 {
                tunnel: [Bits_to_Write."DBS off" ("Bits to write") Bits_to_Write."DBS on" ("Bits to write")] -> w339
                frame False {
                }
                frame True {
                }
              }
              n121 = local read "DO Task"() -> (w340:refnum<k21>)
              n122 = call "WriteDigioBits2_DAQmx.vi"("Bits to write"=w339, "DO Task"=w340) -> ()  [unwired: 9 in, 1 out]
            }
          }
        }
        n123 = local read "Assign settings"() -> (w323:bool)
        n124 = local read "stop"() -> (w334:bool)
        n125 = Wait Until Next ms Multiple(millisecond multiple=u32 150) -> ()  [unwired: 1 out]
        n126 = Or(x="Read Settings", y=w323) -> (x .or. y?=w324:bool)
        n127 = case shown="True" w324 {
          tunnel: w323 -> [_ w398]
          frame False {
          }
          frame True {
            n128 = local read "next trial path"() -> (w399:path)
            n129 = case shown="True" w398 {
              tunnel: [enum16{"Query & Read", "Assign & Read", "Write"}."Assign & Read" ("Read/write") enum16{"Query & Read", "Assign & Read", "Write"}."Query & Read" ("Read/write")] -> w401
              frame True {
                n130 = local write "Assign settings"(FALSE ("Assign settings")) -> ()
              }
              frame False {
              }
            }
            n131 = call "ReadWriteSettingsFile4.vi"("file path"=w399, "Read/write"=w401) -> ("Settings Out"=w419:T5, "current path"=→"current path":path)  [unwired: 4 in, 2 out]
            n132 = Unbundle By Name(w419) -> ("Pre-I hold"=w418:cluster{"Fixed (s)":dbl, "Random (s)":dbl}, "LED I duration"=w417:cluster{"Fixed (s)":dbl, "Random (s)":dbl}, "All Flash?"=w416:bool, "Pre-cue brightness"=w415:i16, "Post-I hold"=w414:cluster{"Fixed (s)":dbl, "Random (s)":dbl}, "Post-I \nbounce-off"=w413:cluster{"Fixed (s)":dbl, "Random (s)":dbl}, "Capture timeout"=w412:cluster{"Fixed (s)":dbl, "Random (s)":dbl}, "Tone duration"=w411:cluster{"Fixed (s)":dbl, "Random (s)":dbl}, "LED C duration"=w410:cluster{"Fixed (s)":dbl, "Random (s)":dbl}, "Cue brightness"=w409:i16, "Hold duration"=w408:cluster{"Fixed (s)":dbl, "Random (s)":dbl}, "Allowed\nbounce-off"=w407:cluster{"Fixed (s)":dbl, "Random (s)":dbl}, "Post-capture brightness"=w406:i16, "Reward duration"=w405:cluster{"Fixed (s)":dbl, "Random (s)":dbl}, "Intertrial interval"=w404:cluster{"Fixed (s)":dbl, "Random (s)":dbl}, "Persistent Mode?"=w403:bool, "Error bong?"=w402:bool, "Critter"=w397:u16, "Target set"=w396:i16[], "Rand/Seq?"=w395:bool, "Trial type"=w394:u16, "Sines?"=w393:bool, "Bumps"=w392:bool, "Sine parameters"=w391:T3, "Bump timing"=w390:cluster{"Fix":dbl, "Rnd":dbl}, "Bump Parameters"=w389:T2, "DBS On?"=w388:bool, "Home reward?"=w387:bool, "Home+target OK?"=w386:bool)
            n133 = local write "Pre-I hold"(w418) -> ()
            n134 = local write "All Flash?"(w416) -> ()
            n135 = local write "Post-I hold"(w414) -> ()
            n136 = local write "Capture timeout"(w412) -> ()
            n137 = local write "LED C duration"(w410) -> ()
            n138 = local write "Hold duration"(w408) -> ()
            n139 = local write "Post-capture brightness"(w406) -> ()
            n140 = local write "Intertrial interval"(w404) -> ()
            n141 = local write "Error\nbong?"(w402) -> ()
            n142 = local write "Target set"(w396) -> ()
            n143 = local write "Trial type"(w394) -> ()
            n144 = local write "Home+target OK?"(w386) -> ()
            n145 = local write "DBS On?"(w388) -> ()
            n146 = local write "Bumps"(w392) -> ()
            n147 = local write "Bump delay"(w390) -> ()
            n148 = local write "Sine parameters"(w391) -> ()
            n149 = local write "Bump Parameters"(w389) -> ()
            n150 = local write "Home reward?"(w387) -> ()
            n151 = local write "Rand/Seq?"(w395) -> ()
            n152 = local write "Persistent\n Mode?"(w403) -> ()
            n153 = local write "LED I duration"(w417) -> ()
            n154 = local write "Pre-cue brightness"(w415) -> ()
            n155 = local write "Post-I \nbounce-off"(w413) -> ()
            n156 = local write "Tone duration"(w411) -> ()
            n157 = local write "Cue brightness"(w409) -> ()
            n158 = local write "Allowed\nbounce-off"(w407) -> ()
            n159 = local write "Reward duration"(w405) -> ()
            n160 = local write "Critter"(w397) -> ()
            n161 = local write "Sines?"(w393) -> ()
          }
        }
        n162 = local read "DI Task"() -> (w332:refnum<k21>)
        n163 = local read "Touch lines"() -> (w331:T7)
        n164 = call "CheckAllTouchSensors.vi"("Touch sensor lines"=w331, "DI Task"=w332) -> ("TS 4"=→"TS 4":bool, "TS 3"=→"TS 3":bool, "TS 2"=→"TS 2":bool, "TS 1"=→"TS 1":bool, "Home?"=→"TS Home":bool)
        n165 = local read "DO Task"() -> (w306:refnum<k21>)
        n166 = call "Control Motor.vi"("Sines?"="Sines?", "Command"=enum16{"Initialize", "Home", "Run", "Disable"}."Run", "Re-center\nmotor"="Recenter motor", "DO Task"=w306, "Sine parameters"="Sine parameters", "Override bumps"="Override bumps", "Home"="Home", "Bumps"="Bumps", "Bump timing"="Bump delay", "Start bump timer?"="Start bump timer?", "Bump Parameters"="Bump Parameters") -> ("Reset\nrecenter"=w308:bool, "Reset override bumps"=w310:bool, "Reset start button"=w312:bool)  [unwired: 2 in]
        n167 = local write "Start bump timer?"(w312) -> ()
        n168 = local write "Recenter motor"(w308) -> ()
        n169 = local write "Override bumps"(w310) -> ()
      }
      n170 = while {
        stop <- w46 stop-if-true
        # "Loop--cycle through all blocks in list until all blocks are completed"
        n171 = stacked-sequence {
          tunnel: [_ _ _ _ w289] -> w49
          tunnel: [_ _ w281 _ _] -> w47
          frame #0 {
            n172 = local read "Exp reset"() -> (w264:bool)
            n173 = case shown="True" w264 {
              frame False {
              }
              frame True {
                n174 = stacked-sequence {
                  frame #0 {
                    n175 = call <vilib>:"Beep.vi"() -> ()  [unwired: 12 in]
                    n176 = Wait (ms)(milliseconds to wait=u32 5) -> ()  [unwired: 1 out]
                  }
                  frame #1 {
                    n177 = local write "Exp reset"(FALSE ("Exp reset")) -> ()
                  }
                  frame #2 {
                    n178 = local write "target set #"(0 ("target set #")) -> ()
                  }
                  frame #3 {
                    n179 = call "TrackStats2.vi"("Command"=T10."Reset for exp") -> ("Total incorrect"=w277:i32, "Total correct"=w276:i32, "# total trials"=w275:i32, "Total % correct"=w274:dbl, "Segment trials"=w273:i32, "Experiment trials"=w270:i32, "Experiment correct"=w268:i32, "Experiment %"=w271:dbl, "Segment Percentage"=w272:dbl)  [unwired: 6 in]
                    n180 = local write "Exp trials"(w270) -> ()
                    n181 = local write "Total incorrect"(w277) -> ()
                    n182 = local write "Total correct"(w276) -> ()
                    n183 = local write "Exp %"(w271) -> ()
                    n184 = local write "Exp correct"(w268) -> ()
                    n185 = local write "Block %"(w272) -> ()
                    n186 = local write "Block trials"(w273) -> ()
                    n187 = local write "Total trials"(w275) -> ()
                    n188 = local write "Total %"(w274) -> ()
                  }
                }
              }
            }
          }
          frame #1 {
            n189 = local read "target set #"() -> (w278:i32)
            n190 = Increment(x=w278) -> (x+1=w279:i32)
            n191 = local write "target set #"(w279) -> ()
          }
          frame #2 {
            n192 = local read "target set #"() -> (w286:i32)
            n193 = call "GetSettingsFileFromTargetSetNum.vi"("target set #"=w286, "# Cycles"="# Cycles", "Block"="Block") -> ("# target sets"=→"# target sets":u16, "Completed list?"=w281:bool, "apply new settings?"=→"Assign settings":bool, "Settings file"=→"next trial path":path)  [unwired: 1 in]
          }
          frame #3 {
            n194 = local read "Assign settings"() -> (w287:bool)
            n195 = case shown="True" w287 {
              frame False {
              }
              frame True {
                # "500ms delay to allow \nsettings loop below to\ninstantiate new settings"
                n196 = Wait (ms)(milliseconds to wait=u32 500) -> ()  [unwired: 1 out]
              }
            }
          }
          frame #4 {
            n197 = call "TargetOverride.vi"("Override 1"="Override 1", "Override 2"="Override 2", "Override 3"="Override 3", "Override 4"="Override 4", "Target set"="Target set") -> ("Target set out"=w295:i16[])  [unwired: 1 in]
            n198 = case shown="True" "Rand/Seq?" {
              tunnel: w295 -> [w299 w301]
              tunnel: [w299 w300] -> w290
              frame False {
              }
              frame True {
                n199 = call "RandomizeTargetSet.vi"("Target set"=w301) -> ("Target set rand order"=w300:i16[])
              }
            }
            n200 = Increment(x=w290) -> (x+1=w289:i16[])
            n201 = Array Size(array=w289) -> (size(s)=→"target set size":i32)
          }
        }
        n202 = local read "stop"() -> (w48:bool)
        n203 = while {
          tunnel: w49 -> [w60] mode=indexing
          tunnel: w49 -> [w59]
          shift-right: [w51] -> _
          shift-left: _ -> [w50]
          i -> [w58]
          stop <- w52 stop-if-true
          # "Loop--do each target in set until target set is completed"
          n204 = Array Size(array=w59) -> (size(s)=w57:i32)
          n205 = Increment(x=w58) -> (x+1=w56:i32)
          n206 = Greater Or Equal?(x=w56, y=w57) -> (x >= y?=w54:bool)
          n207 = local read "stop"() -> (w55:bool)
          n208 = while {
            shift-right: [w70] -> _
            shift-left: T8."Pre-instruction hold init" ("Current stage") -> [w69]
            tunnel: w60 -> [w68]
            shift-right: [w63] -> w51
            shift-left: w50 -> [w62]
            stop <- w65 stop-if-true
            # "Loop--go through each stage of trial until trial is completed"
            n209 = case shown="\"Reward stage\"" w69 {
              tunnel: [T8."Pre-instruction hold" ("Current stage") w81 T8."Instruction" ("Current stage") w131 w140 w153 T8."Target capture" ("Current stage") w175 T8."Target hold" ("Current stage") w195 T8."Intertrial" ("Current stage") T8."Pre-instruction hold init" ("Current stage")] -> w70
              tunnel: [FALSE ("Just initialized\nhold loop?") w79 FALSE ("End of trial") FALSE ("End of trial") FALSE ("End of trial") FALSE ("End of trial") FALSE ("End of trial") FALSE ("End of trial") FALSE ("End of trial") FALSE ("End of trial") FALSE ("End of trial") w248] -> w67
              tunnel: w68 -> [_ _ w97 _ _ _ _ _ _ _ _ _]
              tunnel: [w71 w78 w96 w126 w138 w146 w154 w167 w176 w186 w197 w226] -> w63
              tunnel: w62 -> [w71 w78 w96 w126 w138 w146 w154 w167 w176 w186 _ w226]
              frame "Pre-instruction hold init", Default {
                # "Writ Catch Trial"
                n210 = call "CalculateFixedPlusRandom2.vi"("Component times"="Pre-I hold") -> ("Composite time"=→"Pre-I hold":dbl)  [unwired: 1 in, 1 out]
                "Touching target\nlast time?" <- FALSE ("Touching target\nlast time?")
                "Just initialized\nhold loop?" <- TRUE ("Just initialized\nhold loop?")
              }
              frame "Pre-instruction hold" {
                n211 = case shown="False" "pause" {
                  tunnel: [w92 T8."Pre-instruction hold init" ("Current stage")] -> w81
                  frame False {
                    n212 = local read "Just initialized\nhold loop?"() -> (w87:bool)
                    n213 = local read "Touching target\nlast time?"() -> (w89:bool)
                    n214 = local read "Touch lines"() -> (w90:T7)
                    n215 = local read "Pre-I hold"() -> (w91:dbl)
                    n216 = local read "DO Task"() -> (w83:refnum<k21>)
                    n217 = local read "DI Task"() -> (w82:refnum<k21>)
                    n218 = call "LookForPreInstHold.vi"("Home reward"="Home reward", "Home reward?"="Home reward?", "DI Task"=w82, "Touch lines"=w90, "Touching home\nlast time?"=w89, "Just initialized\nhold loop?"=w87, "Composite time"=w91, "DO Task"=w83) -> ("Touching home\nthis time?"=w88:bool, "Just initialized\nhold loop out?"=w86:bool, "Next stage in trial"=w92:T8)  [unwired: 1 in]
                    n219 = local write "Touching target\nlast time?"(w88) -> ()
                    n220 = local write "Just initialized\nhold loop?"(w86) -> ()
                  }
                  frame True {
                    n221 = while {
                      stop <- w94 continue-if-true
                      n222 = local read "pause"() -> (w94:bool)
                      n223 = Wait (ms)(milliseconds to wait=u32 100) -> ()  [unwired: 1 out]
                    }
                  }
                }
                n224 = local read "Exp reset"() -> (w79:bool)
              }
              frame "Instruction init" {
                n225 = stacked-sequence {
                  tunnel: w97 -> [_ _ w107 w108 _ _ _]
                  frame #0 {
                    n226 = local read "DO Task"() -> (w100:refnum<k21>)
                    n227 = call "WriteDigioBits2_DAQmx.vi"("Bits to write"=Bits_to_Write."In trial on", "DO Task"=w100) -> ()  [unwired: 9 in, 1 out]
                  }
                  frame #1 {
                    n228 = local read "Record flag"() -> (w102:bool)
                    n229 = case shown="True" w102 {
                      frame False {
                      }
                      frame True {
                        n230 = local read "Exp trials"() -> (w106:i32)
                        n231 = local read "DO Task"() -> (w104:refnum<k21>)
                        n232 = Increment(x=w106) -> (x+1=w103:i32)
                        n233 = call "WriteDigioBits2_DAQmx.vi"("Bits to write"=Bits_to_Write."Trial number", "Number"=w103, "DO Task"=w104) -> ()  [unwired: 8 in, 1 out]
                      }
                    }
                  }
                  frame #2 {
                    "Target" <- w107
                  }
                  frame #3 {
                    n234 = local read "DO Task"() -> (w109:refnum<k21>)
                    n235 = call "WriteDigioBits2_DAQmx.vi"("Bits to write"=Bits_to_Write."Target number", "Number"=w108, "DO Task"=w109) -> ()  [unwired: 8 in, 1 out]
                  }
                  frame #4 {
                    n236 = case shown="1" "Trial type" {
                      tunnel: [Bits_to_Write."Trial type preQ off" ("Bits to write") Bits_to_Write."Trial type preQ on" ("Bits to write")] -> w111
                      frame 0, Default {
                        # "Trial type = all flash"
                      }
                      frame 1 {
                        # "Trial type = precue"
                      }
                    }
                    n237 = local read "DO Task"() -> (w112:refnum<k21>)
                    n238 = call "WriteDigioBits2_DAQmx.vi"("Bits to write"=w111, "DO Task"=w112) -> ()  [unwired: 9 in, 1 out]
                  }
                  frame #5 {
                    n239 = call "CalculateFixedPlusRandom2.vi"("Component times"="LED I duration") -> ("Composite time"=w116:dbl)  [unwired: 1 in, 1 out]
                    "Instruct duration" <- w116
                    n240 = Greater Than 0?(x=w116) -> (x > 0?=w117:bool)
                    n241 = case shown="True" w117 {
                      frame False {
                      }
                      frame True {
                        w124 = TRUE  # Initialize?
                        n242 = local read "Pre-cue brightness"() -> (w122:i16)
                        n243 = local read "All Flash?"() -> (w121:bool)
                        n244 = local read "DO Task"() -> (w120:refnum<k21>)
                        n245 = local read "DI Task"() -> (w119:refnum<k21>)
                        n246 = local read "Target"() -> (w123:i16)
                        n247 = call "Instruction.vi"("Initialize?"=w124, "DI Task"=w119, "All Flash?"=w121, "brightness"=w122, "Target"=w123, "DO Task"=w120) -> ()  [unwired: 4 in, 2 out]
                      }
                    }
                  }
                  frame #6 {
                    n248 = local read "Bumps"() -> (w125:bool)
                    n249 = local write "Start bump timer?"(w125) -> ()
                  }
                }
              }
              frame "Instruction" {
                w136 = FALSE  # Initialize?
                n250 = local read "Instruct duration"() -> (w132:dbl)
                n251 = local read "Touch lines"() -> (w137:T7)
                n252 = local read "DO Task"() -> (w128:refnum<k21>)
                n253 = local read "DI Task"() -> (w127:refnum<k21>)
                n254 = local read "Target"() -> (w134:i16)
                n255 = call "Instruction.vi"("Initialize?"=w136, "DI Task"=w127, "All Flash?"="All Flash?", "Touch lines"=w137, "Instruction duration"=w132, "brightness"="Pre-cue brightness", "Target"=w134, "DO Task"=w128) -> ("Last trial successful?"=w135:bool, "Go to stage"=w131:T8)  [unwired: 2 in]
                n256 = local write "Last trial successful?"(w135) -> ()
              }
              frame "Post-instruction hold init" {
                w144 = TRUE  # Initialize?
                # "Writ Catch Trial"
                n257 = local read "DI Task"() -> (w145:refnum<k21>)
                n258 = call "LookForPostInstHold.vi"("Initialize?"=w144, "Post-I \nbounce-off"="Post-I \nbounce-off", "Post-I hold"="Post-I hold", "DI Task"=w145) -> ("Last trial successful?"=w143:bool, "Go to stage"=w140:T8)  [unwired: 6 in]
                n259 = local write "Last trial successful?"(w143) -> ()
              }
              frame "Post-instruction hold" {
                w150 = FALSE  # Initialize?
                # "This is to clear our Catch Boolean during\nthe reward cycle. We put it here so it was\non long enough for us to catch."
                n260 = local read "Touch lines"() -> (w152:T7)
                n261 = local read "DI Task"() -> (w151:refnum<k21>)
                n262 = local write "Catch Trial?"(FALSE) -> ()
                n263 = call "LookForPostInstHold.vi"("Initialize?"=w150, "Touch lines"=w152, "DI Task"=w151) -> ("Last trial successful?"=w149:bool, "Go to stage"=w153:T8)  [unwired: 7 in]
                n264 = local write "Last trial successful?"(w149) -> ()
              }
              frame "Target capture init" {
                w164 = TRUE  # Initialize?
                n265 = local read "DO Task"() -> (w156:refnum<k21>)
                n266 = local read "DI Task"() -> (w155:refnum<k21>)
                n267 = local read "Target"() -> (w162:i16)
                n268 = call "TargetCapture.vi"("DO Task"=w156, "DI Task"=w155, "Response time"="Capture timeout", "Tone duration"="Tone duration", "LED C duration"="LED C duration", "Target"=w162, "Cue brightness"="Cue brightness", "Initialize?"=w164) -> ("Last trial successful?"=w160:bool)  [unwired: 6 in, 1 out]
                n269 = local write "Last trial successful?"(w160) -> ()
              }
              frame "Target capture" {
                w172 = FALSE  # Initialize?
                # "Writ Catch Trial"
                n270 = local read "Target"() -> (w166:i16)
                n271 = local read "Touch lines"() -> (w173:T7)
                n272 = local read "DO Task"() -> (w169:refnum<k21>)
                n273 = local read "DI Task"() -> (w168:refnum<k21>)
                n274 = call "TargetCapture.vi"("DO Task"=w169, "Touch lines"=w173, "DI Task"=w168, "Home+target OK?"="Home+target OK?", "Target"=w166, "Initialize?"=w172) -> ("Go to stage"=w175:T8, "Last trial successful?"=w174:bool)  [unwired: 8 in]
                n275 = local write "Last trial successful?"(w174) -> ()
              }
              frame "Target hold init" {
                w182 = TRUE  # Initialize?
                n276 = local read "DO Task"() -> (w178:refnum<k21>)
                n277 = local read "DI Task"() -> (w177:refnum<k21>)
                n278 = local read "Target"() -> (w180:i16)
                n279 = call "TargetHold.vi"("DO Task"=w178, "DI Task"=w177, "target hold"="Hold duration", "target\nbounce-off"="Allowed\nbounce-off", "Target"=w180, "Post-capture brightness"="Post-capture brightness", "Initialize?"=w182) -> ()  [unwired: 7 in, 2 out]
              }
              frame "Target hold" {
                w190 = FALSE  # Initialize?
                n280 = local read "Home+target OK?"() -> (w188:bool)
                n281 = local read "Touch lines"() -> (w193:T7)
                n282 = local read "DO Task"() -> (w194:refnum<k21>)
                n283 = local read "DI Task"() -> (w187:refnum<k21>)
                n284 = local read "Target"() -> (w192:i16)
                n285 = call "TargetHold.vi"("DO Task"=w194, "Touch lines"=w193, "DI Task"=w187, "Home+target OK?"=w188, "Target"=w192, "Initialize?"=w190) -> ("Go to stage"=w195:T8, "Last trial successful?"=w191:bool)  [unwired: 8 in]
                n286 = local write "Last trial successful?"(w191) -> ()
              }
              frame "Reward stage" {
                n287 = flat-sequence {
                  tunnel: [w204] -> w196
                  tunnel: [w221] -> w197
                  tunnel: w196 -> [w221]
                  frame #0 {
                    n288 = Random Number (0-1)() -> (number: 0 to 1=w211:dbl)
                    n289 = Multiply(x=w211, y=100.0) -> (x*y=w210:dbl)
                    n290 = To Unsigned Long Integer(number=w210) -> (unsigned 32bit integer=w209:u32)
                    n291 = Less Or Equal?(x=w209, y="Catch probability") -> (x <= y?=w202:bool)
                    n292 = Not Equal To 0?(x="Catch probability") -> (x != 0?=w201:bool)
                    n293 = And(x=w201, y=w202) -> (x .and. y?=w200:bool)
                    n294 = case shown="True" w200 {
                      selector: w200 -> [w216 w218]
                      tunnel: ["Reward duration" cluster{"Fix":dbl, "Rnd":dbl} {"Fix"=0.0, "Rnd"=0.0} ("Reward duration")] -> w214
                      tunnel: [w216 w218] -> w204
                      frame False {
                        # "Sending False bit for \ncatch trial"
                        # "Normal reward duration"
                      }
                      frame True {
                        # "Sending True bit for \ncatch trial"
                        # "This is the catch trial. \nSo we don't want to deliver \na reward"
                      }
                    }
                    "Catch Trial?" <- w204
                    n295 = call "CalculateFixedPlusRandom2.vi"("Component times"=w214) -> ("time in ms"=w215:dbl)  [unwired: 1 in, 1 out]
                    n296 = local read "DO Task"() -> (w213:refnum<k21>)
                    n297 = call "Reward Pulse.vi"("Pulse duration (ms)"=w215, "DO Task"=w213) -> ()  [unwired: 8 in]
                    n298 = Select(t=Bits_to_Write."LED 4 on" ("Bits to write"), s=w204, f=Bits_to_Write."LED 4 off" ("Bits to write")) -> (s? t:f=w205:T9)
                    n299 = call "WriteDigioBits2_DAQmx.vi"("Bits to write"=w205, "DO Task"=refnum<k21> "BlueSimple_DO_All" ("DO Task 2")) -> ()  [unwired: 9 in, 1 out]
                  }
                  frame #1 {
                    # "This second sequence is for the Arm Freeze Reward Timer.\nWhen the monkey reaches to the target, her arm freezes.\nThis routine provides a timer to notify the tirainer to give \nthe monkey a treat and return her arm to the home key."
                    n300 = case shown="True" "Arm Freeze Counter" {
                      frame False {
                      }
                      frame True {
                        n301 = flat-sequence {
                          frame #0 {
                            n302 = Multiply(x="Time to wait\nbefore treat \nArm freeze (S)", y=1000) -> (x*y=w222:dbl)
                            n303 = Wait (ms)(milliseconds to wait=w222) -> ()  [unwired: 1 out]
                          }
                          frame #1 {
                            n304 = call <vilib>:"Beep.vi"("use system alert? (T)"=TRUE) -> ()  [unwired: 11 in]
                          }
                        }
                      }
                    }
                  }
                }
              }
              frame "Intertrial" {
                n305 = local read "Last trial successful?"() -> (w244:bool)
                n306 = local read "target set size"() -> (w232:i32)
                n307 = local read "# target sets"() -> (w233:u16)
                n308 = local read "Bumps"() -> (w228:bool)
                n309 = Multiply(x=w233, y=w232) -> (x*y=w231:i32)
                n310 = local write "Override bumps"(w228) -> ()
                n311 = local write "Recenter motor"(w228) -> ()
                n312 = call "TrackStats2.vi"("Last trial successful?"=w244, "Trial bin size"=w231, "Persistent\n Mode?"="Persistent\n Mode?", "Command"=enum16{"Reset", "Increment"}."Increment") -> ("Total incorrect"=→"Total incorrect":i32, "Total correct"=→"Total correct":i32, "# total trials"=→"Total trials":i32, "Total % correct"=w236:dbl, "Segment trials"=→"Block trials":i32, "Experiment trials"=→"Exp trials":i32, "Experiment correct"=→"Exp correct":i32, "Experiment %"=→"Exp %":dbl, "Segment Percentage"=w237:dbl)  [unwired: 3 in]
                "Block %" <- w237
                "Total %" <- w236
                n313 = Bundle("Segment Percentage"=w237, "Total % correct"=w236) -> (→"Waveform Chart":T6)  [unwired: 1 in]
                n314 = call "CalculateFixedPlusRandom2.vi"("Component times"="Intertrial interval") -> ("Composite time"=w245:dbl)  [unwired: 1 in, 1 out]
                n315 = while {
                  shift-right: [enum16{"Start counting", "Read count", "Reset"}."Read count" ("Enum")] -> _
                  shift-left: enum16{"Start counting", "Read count", "Reset"}."Start counting" ("Enum") -> [w263]
                  tunnel: [w258] -> _
                  tunnel: w245 -> [w257]
                  stop <- w259 stop-if-true
                  n316 = call "non-Reentrant Controllable Timer.vi"("Enum"=w263) -> ("Time out"=w261:dbl)  [unwired: 1 in]
                  n317 = local read "stop"() -> (w260:bool)
                  n318 = Greater Or Equal?(x=w261, y=w257) -> (x >= y?=w258:bool)
                  n319 = Or(x=w258, y=w260) -> (x .or. y?=w259:bool)
                }
                n320 = local read "Persistent\n Mode?"() -> (w234:bool)
                n321 = case shown="False" w234 {
                  tunnel: [w255 w256] -> w248
                  frame False {
                    w255 = TRUE  # End of trial
                  }
                  frame True {
                    n322 = local read "Last trial successful?"() -> (w256:bool)
                  }
                }
                n323 = stacked-sequence {
                  frame #0 {
                    n324 = local read "Last trial successful?"() -> (w250:bool)
                    n325 = case shown="False" w250 {
                      frame False {
                        n326 = local read "DO Task"() -> (w251:refnum<k21>)
                        n327 = call "Signal Error.vi"("DO Task"=w251, "Error bong?"="Error\nbong?") -> ()  [unwired: 3 in]
                      }
                      frame True {
                      }
                    }
                  }
                  frame #1 {
                    n328 = local read "DO Task"() -> (w253:refnum<k21>)
                    n329 = call "WriteDigioBits2_DAQmx.vi"("Bits to write"=Bits_to_Write."In trial off", "DO Task"=w253) -> ()  [unwired: 9 in, 1 out]
                  }
                  frame #2 {
                  }
                }
              }
            }
            n330 = Wait (ms)(milliseconds to wait=u32 1) -> ()  [unwired: 1 out]
            n331 = Compound Arithmetic op=OR(w67, "stop") -> (w65:bool)
            "Current stage" <- w69
          }
          n332 = local read "Exp reset"() -> (w53:bool)
          n333 = Compound Arithmetic op=OR(w55, w54, w53) -> (w52:bool)
        }
        n334 = Or(x=w48, y=w47) -> (x .or. y?=w46:bool)
      }
    }
    frame #3 {
      # "Turn LED's, \nbuzzer,\npump off\njust to be\nsure"
      n335 = local read "DO Task"() -> (w436:refnum<k21>)
      n336 = local read "DO Task"() -> (w434:refnum<k21>)
      n337 = local read "DO Task"() -> (w438:refnum<k21>)
      n338 = local read "DO Task"() -> (w439:refnum<k21>)
      n339 = local read "DO Task"() -> (w441:refnum<k21>)
      n340 = local read "DO Task"() -> (w443:refnum<k21>)
      n341 = local write "Record flag"(FALSE ("Record flag")) -> ()
      n342 = call "WriteDigioBits2_DAQmx.vi"("Bits to write"=Bits_to_Write."In trial off", "DO Task"=w436) -> ()  [unwired: 9 in, 1 out]
      n343 = call "WriteDigioBits2_DAQmx.vi"("Bits to write"=Bits_to_Write."All LEDs off", "DO Task"=w434) -> ()  [unwired: 9 in, 1 out]
      n344 = call "WriteDigioBits2_DAQmx.vi"("Bits to write"=Bits_to_Write."Buzzer off", "DO Task"=w438) -> ()  [unwired: 9 in, 1 out]
      n345 = call "WriteDigioBits2_DAQmx.vi"("Bits to write"=Bits_to_Write."Reward off", "DO Task"=w439) -> ()  [unwired: 9 in, 1 out]
      n346 = call "WriteDigioBits2_DAQmx.vi"("Bits to write"=Bits_to_Write."Error off", "DO Task"=w441) -> ()  [unwired: 9 in, 1 out]
      n347 = call "WriteDigioBits2_DAQmx.vi"("Bits to write"=Bits_to_Write."DBS off", "DO Task"=w443) -> ()  [unwired: 9 in, 1 out]
      n348 = local write "stop"(FALSE ("stop")) -> ()
    }
  }
